vi "dfd_Validate Subband Filters.vi"(8 "error in (no error)":errorcluster, 10 "filter bank structure":T2 items=["Uniform", "Non-Uniform"], 11 "subband filters in":T3[](array[typedef]) {"mMRate_SumWl" min=1 max=32 step=1; "mMRate_InputIwl" min=1 max=32 step=1; "mMRate_GainWl" min=1 max=32 step=1; "mMRate_OutputWl" min=1 max=32 step=1; "mMRate_InputWl" min=1 max=32 step=1; "mMRate_CoefWl" min=1 max=32 step=1; "mMRate_Mode" items=["Default"=-1, "No Rate Change"=0, "Interpolation"=1, "Decimation"=2, "Interpolated"=3, "Rational"=4]}) -> (0 "error out":errorcluster, 1 "filter mode":T1 items=["Default"=-1, "No Rate Change"=0, "Interpolation"=1, "Decimation"=2, "Interpolated"=3, "Rational"=4], 2 "is Valid?":bool, 3 "subband filters out":T3[](array[typedef]) {"mMRate_SumWl" min=1 max=32 step=1; "mMRate_InputIwl" min=1 max=32 step=1; "mMRate_GainWl" min=1 max=32 step=1; "mMRate_OutputWl" min=1 max=32 step=1; "mMRate_InputWl" min=1 max=32 step=1; "mMRate_CoefWl" min=1 max=32 step=1; "mMRate_Mode" items=["Default"=-1, "No Rate Change"=0, "Interpolation"=1, "Decimation"=2, "Interpolated"=3, "Rational"=4]})   [LabVIEW 2017, in "NI_DigFilter_FilterBank.lvlib"]
uses:
  <vilib>/addons/Digital Filter Design/NI_DigFilter_FilterBank.lvlib
  <vilib>/addons/Digital Filter Design/_Objects.llb/DFD Multirate Filter Obj.ctl
  <vilib>/addons/Digital Filter Design/_Objects.llb/DFD Multirate Mode.ctl
  <vilib>/addons/Digital Filter Design/_Objects.llb/DFD Coef Norm Type.ctl
  <vilib>/addons/Digital Filter Design/_Objects.llb/DFD Round-off Mode.ctl
  <vilib>/addons/Digital Filter Design/_Objects.llb/DFD FXP MRate Multiply Mode.ctl
  <vilib>/addons/Digital Filter Design/FilterBank.llb/Object/DFD Filter Bank Type.ctl
  <vilib>/addons/Digital Filter Design/_Objects.llb/DFD Multirate Rational Factor.ctl
  <vilib>/addons/Digital Filter Design/_Misc.llb/dfd_Error Handlers (Single).vi
  <vilib>/addons/Digital Filter Design/NI_DigFilterLicensed.lvlib
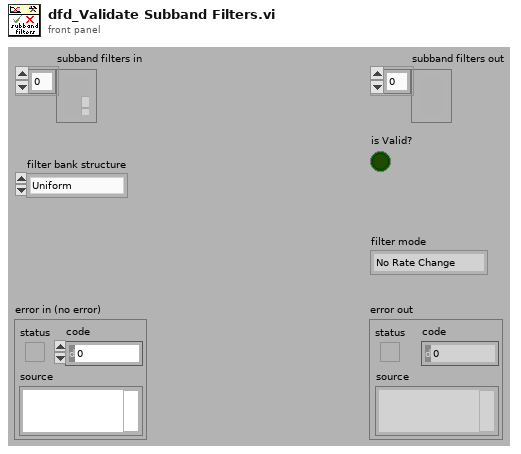
[diagram p1: front panel]
types:
  T1 = typedef "NI_DigFilterLicensed.lvlib/DFD Multirate Mode.ctl" = i16
  T2 = typedef "NI_DigFilter_FilterBank.lvlib/DFD Filter Bank Type.ctl" = u16
  T3 = typedef "NI_DigFilterLicensed.lvlib/DFD Multirate Filter Obj.ctl" = cluster{"mMRate_Structure":enum16{"CIC", "FIR", "IIR", "Lattice"}, "mMRate_Mode":T1, "mMRate_Factor":i32, "mMRate_FIRParams":cluster{"mMRate_FIR_H":dbl[], "mMRate_FIR_IsNyquist?":bool, "mMRate_FIR_IsSymmetric?":bool}, "mMRate_CICParams":cluster{"mMRate_CIC_#Stage":i32, "mMRate_CIC_Lag":i32, "mMRate_CIC_Type":enum16{"Lowpass", "Highpass"}}, "mMRate_Order":i32, "mMRate_Version":string, "mMRate_Comments":string, "mMRate_RationalFactor":cluster{"mMRate_L":i32, "mMRate_M":i32}, "mMRate_Fs":dbl, "mMRate_Quantized?":bool, "mMRate_QFilterGain":dbl, "mMRate_CoefWl":i16, "mMRate_Scaling":cluster{"mMRate_ScaleByPowerOf2?":bool, "mMRate_ScaleType":T4}, "mMRate_InputWl":i16, "mMRate_OutputWl":i16, "mMRate_OutputMode":T5, "mMRate_MultMode":T6, "mMRate_BitPruning":bool, "mMRate_GainWl":i16, "mMRate_OutputFwl":i16, "mMRate_SumIwl":i16, "mMRate_InputIwl ":i16, "mMRate_SumWl":i16, "mMRate_CoefIwl":i16}
  T4 = typedef "NI_DigFilterLicensed.lvlib/DFD Coef Norm Type.ctl" = enum16{"No Norm", "Time Domain 1-Norm", "Time Domain 2-Norm", "Time Domain Inf-Norm"}
  T5 = typedef "NI_DigFilterLicensed.lvlib/DFD Round-off Mode.ctl" = enum16{"Nearest", "Truncation"}
  T6 = typedef "NI_DigFilterLicensed.lvlib/DFD FXP MRate Multiply Mode.ctl" = enum16{"Truncated", "Full"}
  T7 = typedef "NI_DigFilterLicensed.lvlib/DFD Multirate Rational Factor.ctl" = cluster{"L":i32, "M":i32}
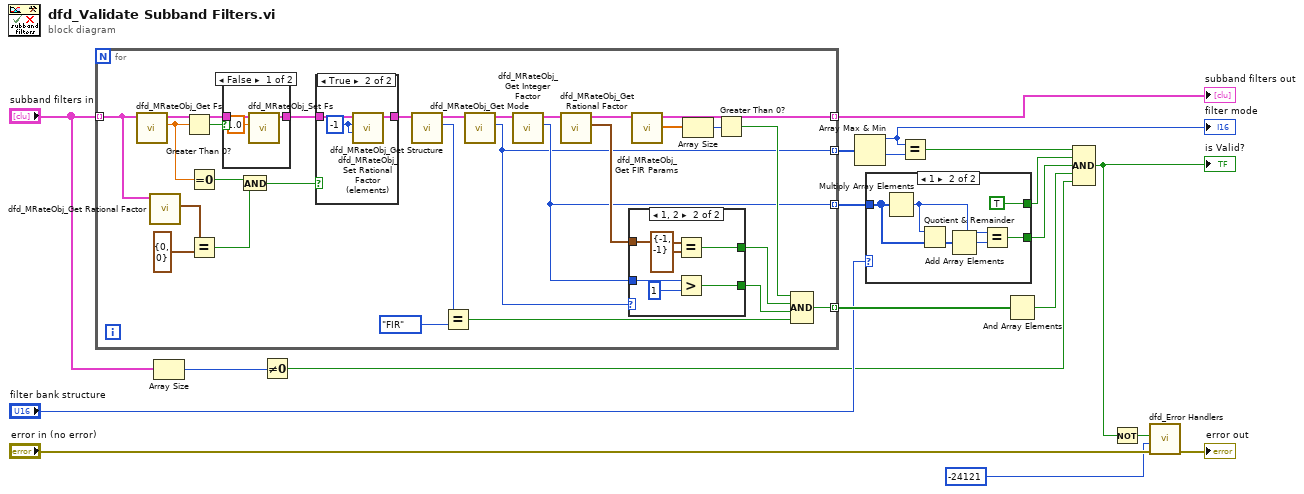
[diagram p0: block diagram]
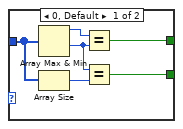
[diagram p2: hidden frame]
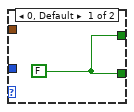
[diagram p3: hidden frame]
diagram:
  n1 = for {
    tunnel: "subband filters in" -> [w24] mode=indexing
    tunnel: [w21] -> w12 mode=indexing
    tunnel: [w23] -> w14 mode=indexing
    tunnel: [w22] -> w9 mode=indexing
    tunnel: [w20] -> w15 mode=indexing
    n2 = call <vilib>:"dfd_MRateObj_Get Fs.vi"("multirate filter in"=w24) -> ("fs"=w35:dbl, "dup multirate filter"=w32:T3)  [unwired: 9 out]
    n3 = call <vilib>:"dfd_MRateObj_Get Rational Factor.vi"("multirate filter in"=w24) -> ("rational factor"=w33:T7)  [unwired: 10 out]
    n4 = Greater Than 0?(x=w35) -> (x > 0?=w31:bool)
    n5 = Equal To 0?(x=w35) -> (x = 0?=w36:bool)
    n6 = Equal?(x=w33, y=T7 {"L"=0, "M"=0}) -> (x = y?=w37:bool)
    n7 = case shown="False" w31 {
      tunnel: w32 -> [w61 w62]
      tunnel: [w60 w62] -> w39
      frame False {
        n8 = call <vilib>:"dfd_MRateObj_Set Fs.vi"("fs"=1.0, "multirate filter in"=w61) -> ("dup multirate filter"=w60:T3)  [unwired: 9 out]
      }
      frame True {
      }
    }
    n9 = And(x=w36, y=w37) -> (x .and. y?=w38:bool)
    n10 = case shown="True" w38 {
      tunnel: w39 -> [w55 w58]
      tunnel: [w55 w57] -> w40
      frame False {
      }
      frame True {
        w56 = -1 ("L")
        n11 = call <vilib>:"dfd_MRateObj_Set Rational Factor (elements).vi"("M"=w56, "L"=w56, "multirate filter in"=w58) -> ("multirate filter out"=w57:T3)  [unwired: 8 out]
      }
    }
    n12 = call <vilib>:"dfd_MRateObj_Get Structure.vi"("multirate filter in"=w40) -> ("structure"=w27:enum16{"CIC", "FIR", "IIR", "Lattice"}, "dup multirate filter"=w25:T3)  [unwired: 9 out]
    n13 = Equal?(x=w27, y=enum16{"CIC", "FIR", "IIR", "Lattice"}."FIR" ("preferred structure")) -> (x = y?=w29:bool)
    n14 = call <vilib>:"dfd_MRateObj_Get Mode.vi"("multirate filter in"=w25) -> ("mode"=w21:T1, "dup multirate filter"=w26:T3)  [unwired: 9 out]
    n15 = call <vilib>:"dfd_MRateObj_Get Integer Factor.vi"("multirate filter in"=w26) -> ("factor"=w22:i32, "dup multirate filter"=w30:T3)  [unwired: 9 out]
    n16 = call <vilib>:"dfd_MRateObj_Get Rational Factor.vi"("multirate filter in"=w30) -> ("rational factor"=w42:T7, "dup multirate filter"=w43:T3)  [unwired: 9 out]
    n17 = case shown="1, 2" w21 {
      tunnel: w22 -> [_ w50]
      tunnel: w42 -> [_ w54]
      tunnel: [w48 w51] -> w45
      tunnel: [w48 w52] -> w46
      frame 0, Default {
        w48 = FALSE
      }
      frame 1, 2 {
        n18 = Equal?(x=w54, y=T7 {"L"=-1, "M"=-1}) -> (x = y?=w52:bool)
        n19 = Greater?(x=w50, y=1) -> (0:w51:bool)
      }
    }
    n20 = call <vilib>:"dfd_MRateObj_Get FIR Params.vi"("multirate filter in"=w43) -> ("h(n)"=w44:dbl[], "dup multirate filter"=w20:T3)  [unwired: 9 out]
    n21 = Array Size(array=w44) -> (size(s)=w41:i32)
    n22 = Greater Than 0?(x=w41) -> (x > 0?=w47:bool)
    n23 = Compound Arithmetic op=AND(w47, w46, w45, w29) -> (w23:bool)
  }
  "subband filters out" <- w15
  n24 = Array Size(array="subband filters in") -> (size(s)=w2:i32)
  n25 = Not Equal To 0?(x=w2) -> (x != 0?=w1:bool)
  n26 = Array Max & Min(array=w12) -> (max value=w11:T1, min value=w10:T1)  [unwired: 2 out]
  "filter mode" <- w11
  n27 = case shown="1" "filter bank structure" {
    tunnel: w9 -> [w66 w73]
    tunnel: [w67 TRUE] -> w7
    tunnel: [w63 w69] -> w6
    frame 0, Default {
      n28 = Array Max & Min(array=w66) -> (max value=w68:i32, min value=w64:i32)  [unwired: 2 out]
      n29 = Array Size(array=w66) -> (size(s)=w65:i32)
      n30 = Equal?(x=w68, y=w64) -> (x = y?=w67:bool)
      n31 = Equal?(x=w64, y=w65) -> (x = y?=w63:bool)
    }
    frame 1 {
      n32 = Multiply Array Elements(1:w73) -> (0:w70:i32)
      n33 = Quotient & Remainder(x=w70, y=w73) -> (floor(x/y)=w72:i32[])  [unwired: 1 out]
      n34 = Add Array Elements(numeric array=w72) -> (sum=w71:i32)
      n35 = Equal?(x=w70, y=w71) -> (x = y?=w69:bool)
    }
  }
  n36 = Equal?(x=w11, y=w10) -> (x = y?=w8:bool)
  n37 = And Array Elements(Boolean array=w14) -> (logical AND=w5:bool)
  n38 = Compound Arithmetic op=AND(w8, w7, w6, w5, w1) -> (w4:bool)
  "is Valid?" <- w4
  n39 = Not(x=w4) -> (.not. x?=w17:bool)
  n40 = call-poly <vilib>:"dfd_Error Handlers.vi"("error in (no error)"="error in (no error)", "error code"=-24121 ("ERR_INVALID_FILTERBANK_OBJ"), "condition failed?"=w17) -> ("error out"=→"error out":errorcluster)  [unwired: 8 out]
